vi "Red Pitaya OO Control.vi"(8 "Error In":errorcluster, 10 "Server port":u16=1002, 11 "Server address":string="192.168.1.100") -> (0 "Error Out":errorcluster)   [LabVIEW 2015]
uses:
  Mode.ctl
  Red Pitaya Parameters.ctl
  RP Core/RP Communicator/RP Communicator.lvclass
  RP Core/RP Communicator/RP Communicator.lvclass/RP Communicator.ctl
  RP Status Offsets.ctl
  RP Command.ctl
  RP Config Offsets.ctl
  RP Core/RP Communicator/Write Client type.vi
panel:
  in  "Controls":enum32{"Basic", "Advanced"}(tab)=enum."Advanced"
  out "X&Y":cluster{i32, i32}(graph)
  in  "Parameters":T1={"Ranges"=[0.0001, 0.01], "Output frequency 1"=15625000.0, "Output frequency 2"=50000.0, "Pre-trigger samples"=-100000, "Post-trigger samples"=11534336, "Desimation rate"=1, "Delayed start"=571428} {"Delayed start" format="0x%x (%d)"; "Post-trigger samples" format="0x%x (%d)"; "Pre-trigger samples" format="0x%x (%d)"; "Output frequency 2" format="%#_6p"; "Output frequency 1" format="%#_6p"; "Ranges" format="%#_12p"}
  out "CPU Temperature":dbl(slide)=48.847186279148 scale=0.0..100.0
  out "Y":i32=1717987 format="0x%x (%d)"
  out "X":i32=1717987 format="0x%x (%d)"
  in  "Read XY":bool
  in  "Trigger pos acuracy":i32=1
  in  "Signal bits":i32=14
  in  "Read Temperature":bool
  in  "Read trigger":bool=TRUE
  in  "Auto-save file":bool
  in  "Samples to read":u64=67108864 format="0x%x (%d)"
  in  "Record":bool
  out "Temperature Chart":dbl(graph)=48.847186279148
  out "bytes written":i32=8
  in  "Status":bool
  out "Status response":u32=1 format="0x%x (%d)"
  out "element":u32
  in  "Status offset":u64=12
  out "Phase increment 1":u64=1717987 format="0x%x (%d)"
  in  "Read":bool
  in  "Send \"Connect client\"":bool=TRUE
  in  "Bytes per sample":i32=4
  out "Is Red Pitaya?":bool
  out "Logic tag out":u16
  out "IDN response":u32=1 format="0x%x (%d)"
  in  "Read subset":bool
  out "Data File  Path":path
  out "Trigger state":bool
  in  "Trigger":bool
  in  "Arm":bool
  out "Phase  Graph":u32[](graph)
  in  "Mode":T2=enum."Current-Voltage"
  out "Waveform Graph":sgl[][](graph)
  in  "Stop Server":bool
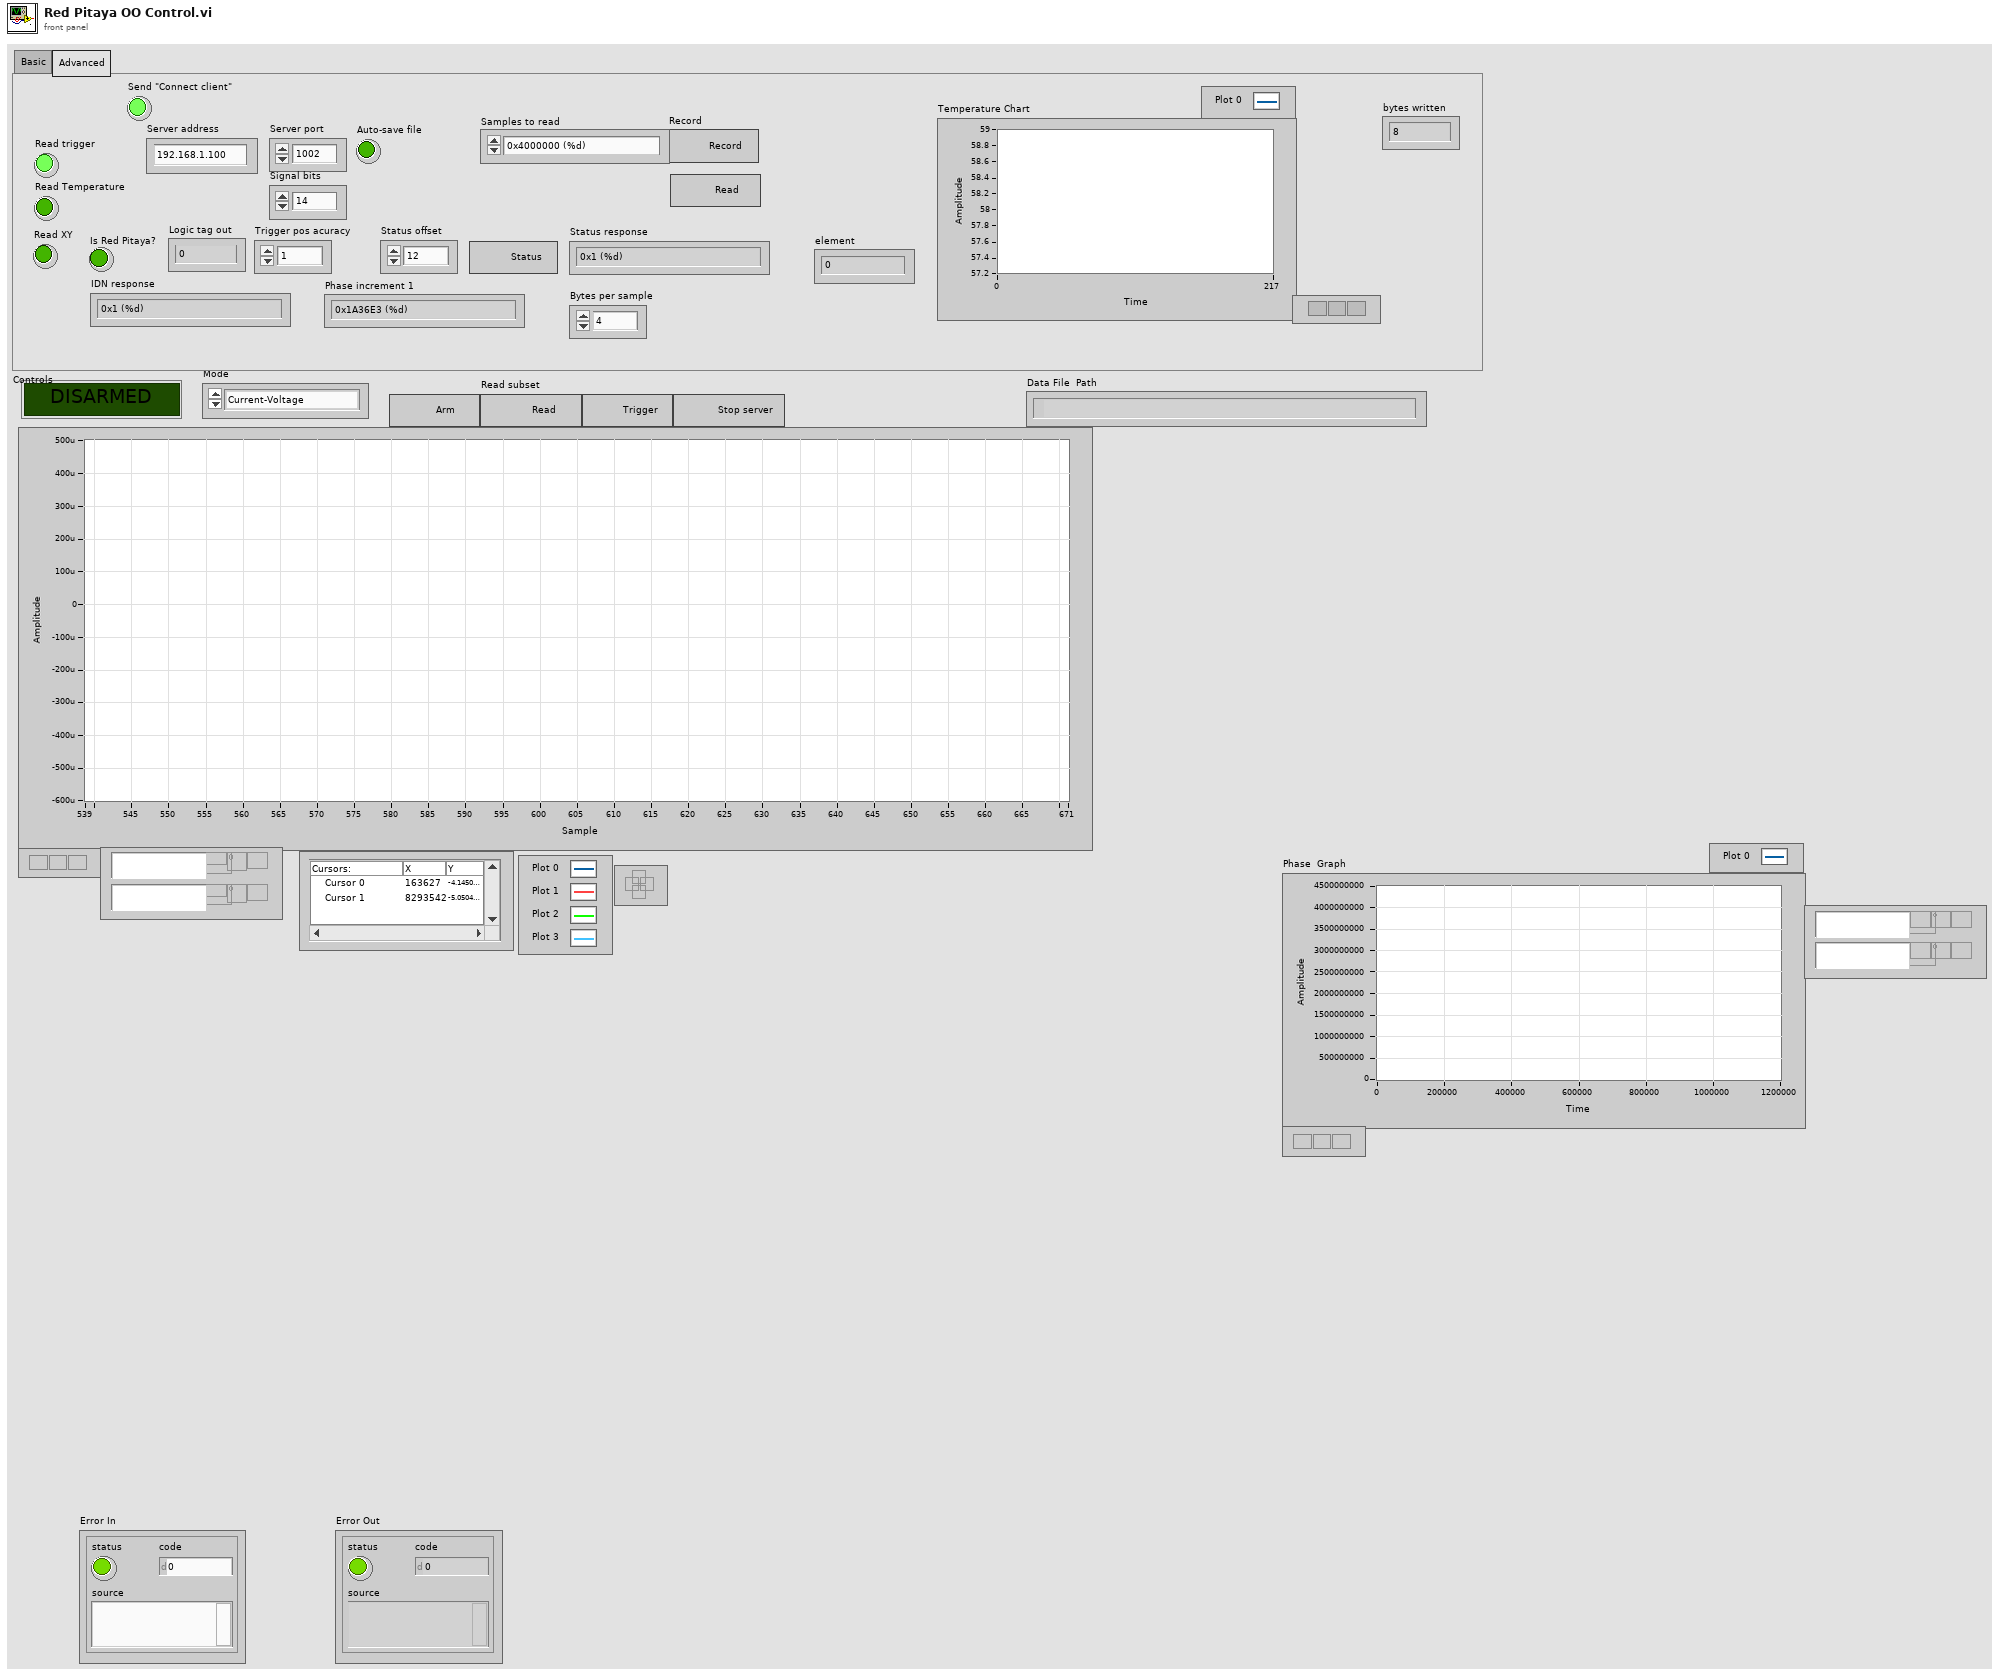
[diagram p1: front panel]
types:
  T1 = typedef "Red Pitaya Parameters.ctl" = cluster{"Ranges":dbl[], "Output frequency 1":dbl, "Output frequency 2":dbl, "Pre-trigger samples":i32, "Post-trigger samples":u64, "Desimation rate":u64, "Delayed start":u64}
  T2 = typedef "Mode.ctl" = enum16{"Filter", "Lockin test", "Snapshot test", "Digitizer", "Current-Voltage"}
  T3 = typedef "RP Command.ctl" = enum16{"Reset", "Read IDN", "Stop server", "Get status", "Get temperature", "Connect client", "Arm", "Software trigger", "Get whole buffer", "Get chunk", "System call", "Get config", "Set config", "Recieve data", "Play pattern", "Transmit data"}
  T4 = typedef "RP Status Offsets.ctl" = u16
  T5 = typedef "RP Config Offsets.ctl" = u16
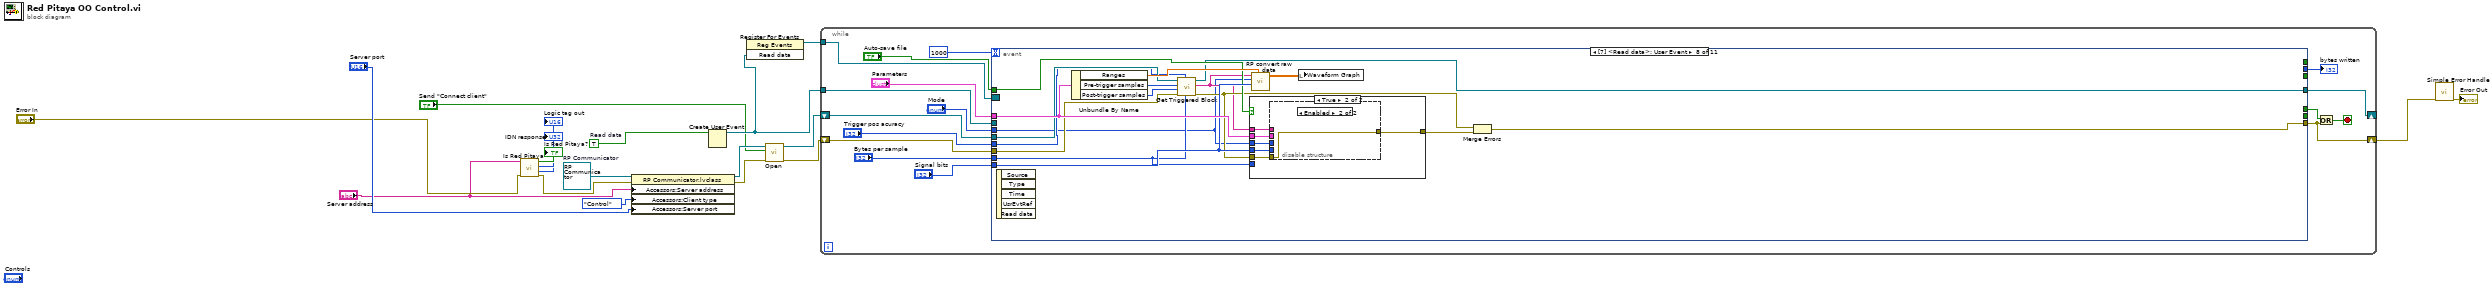
[diagram p0: block diagram]
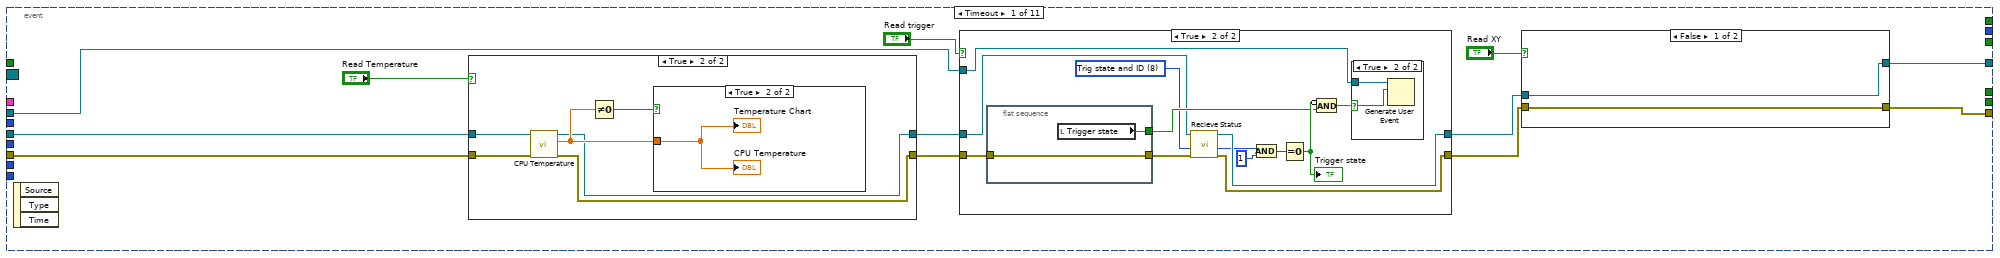
[diagram p2: hidden frame]
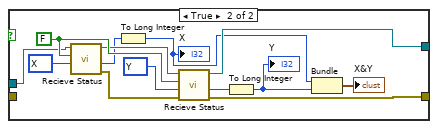
[diagram p3: hidden frame]
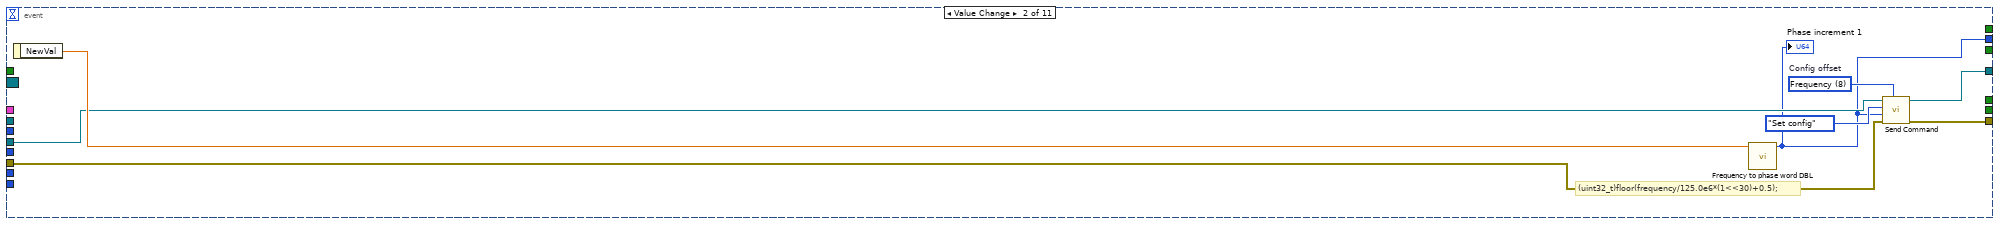
[diagram p8: hidden frame]
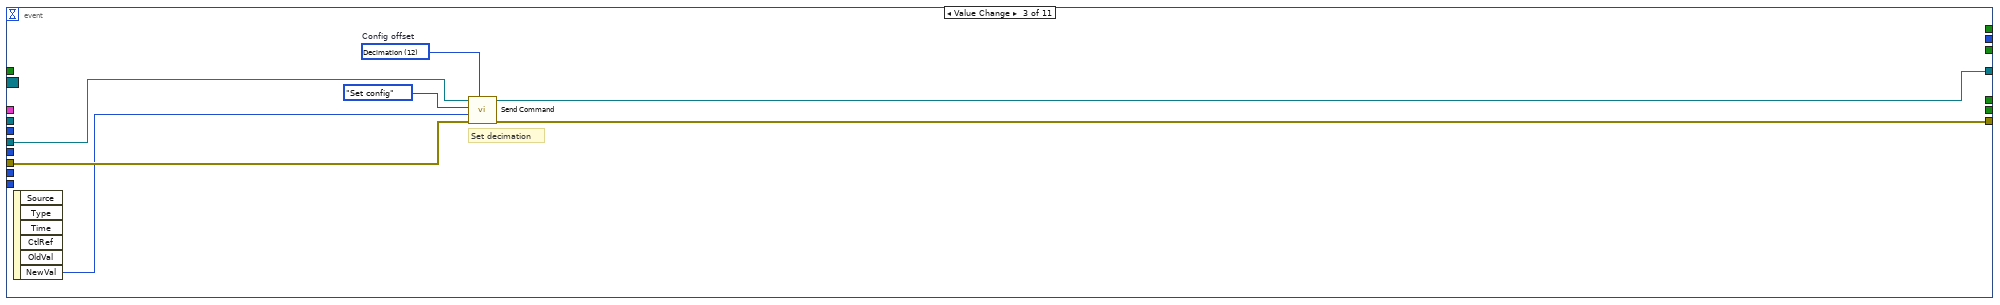
[diagram p9: hidden frame]
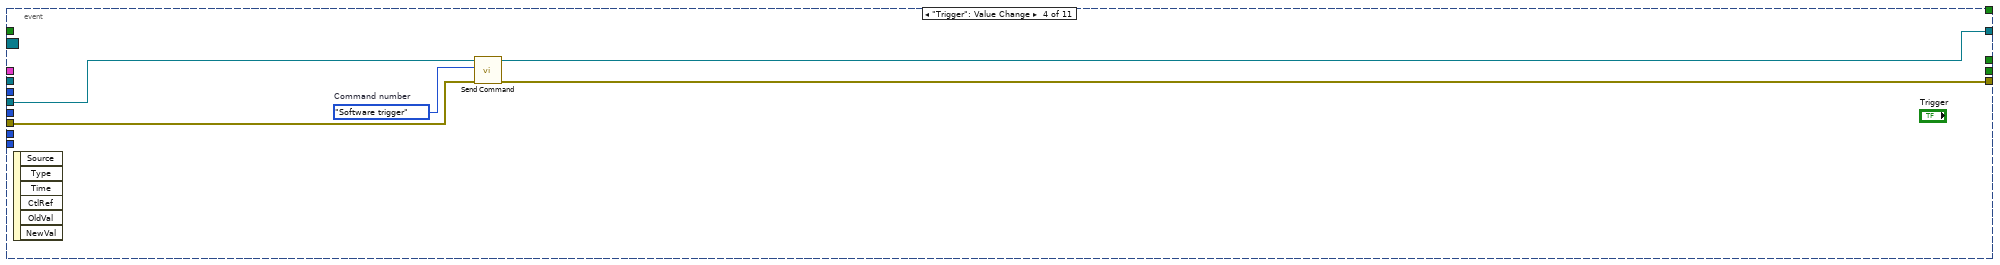
[diagram p10: hidden frame]
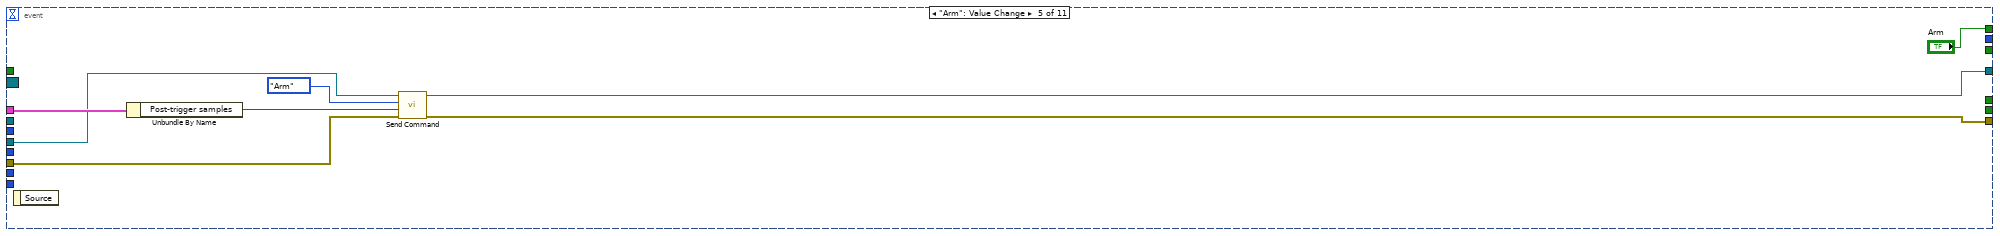
[diagram p11: hidden frame]
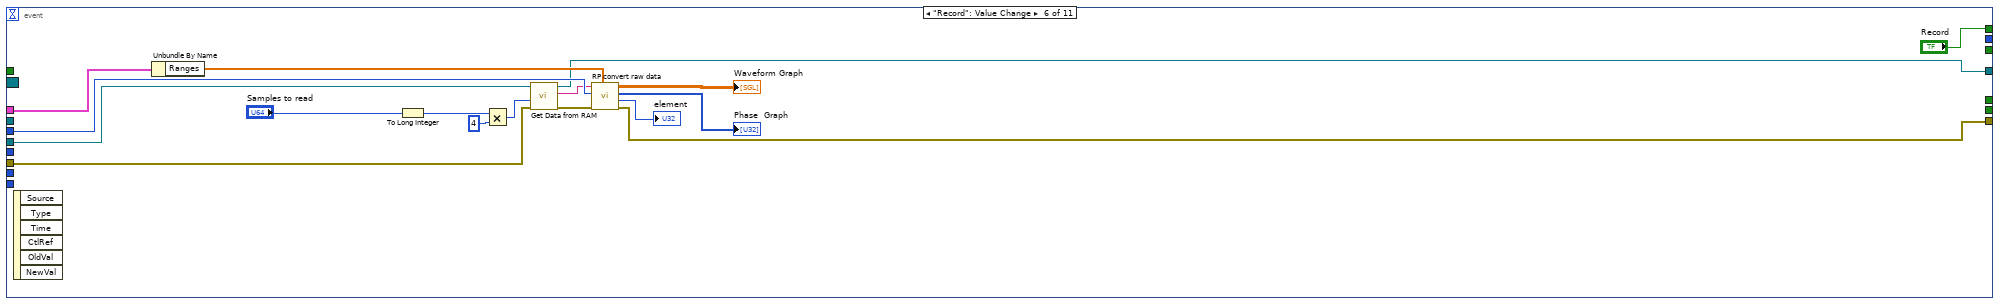
[diagram p12: hidden frame]
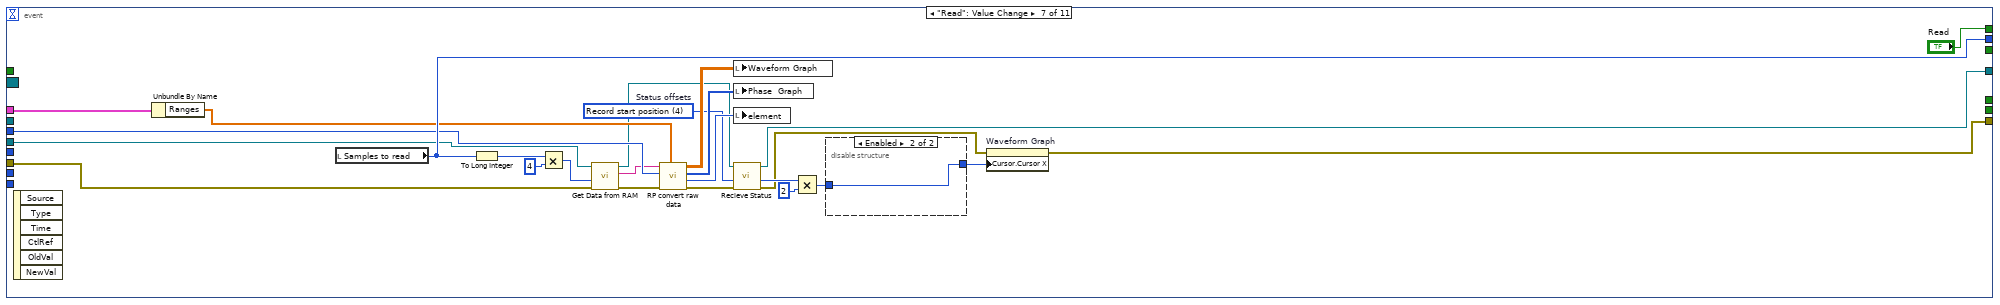
[diagram p13: hidden frame]
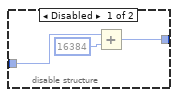
[diagram p14: hidden frame]
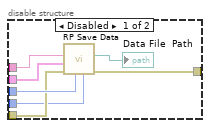
[diagram p16: hidden frame]
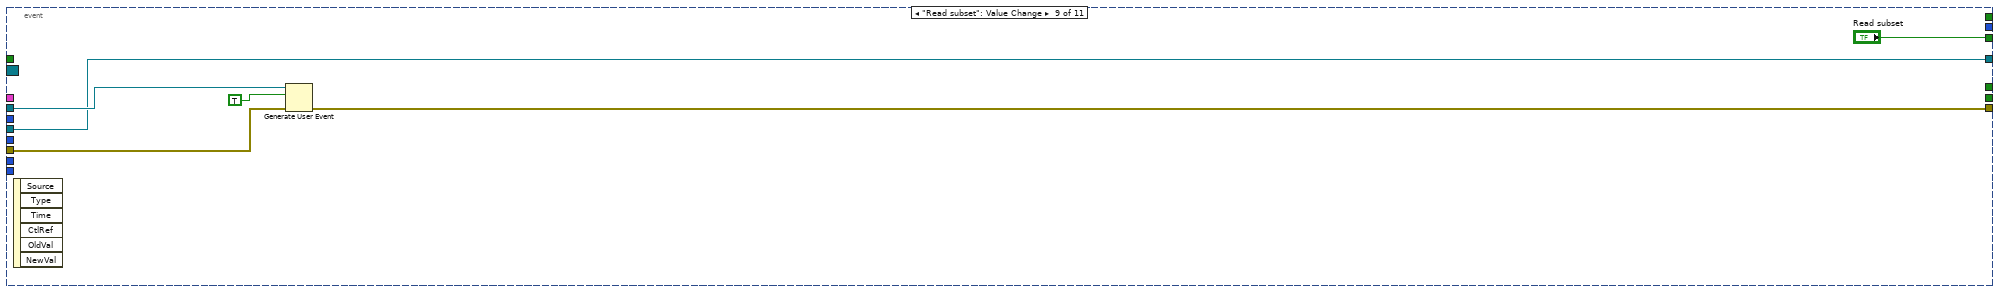
[diagram p17: hidden frame]
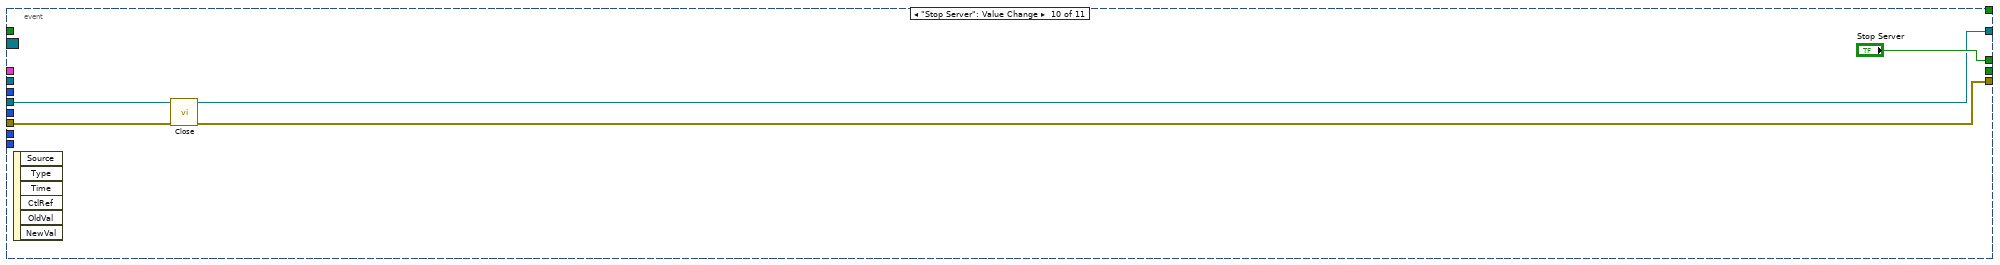
[diagram p18: hidden frame]
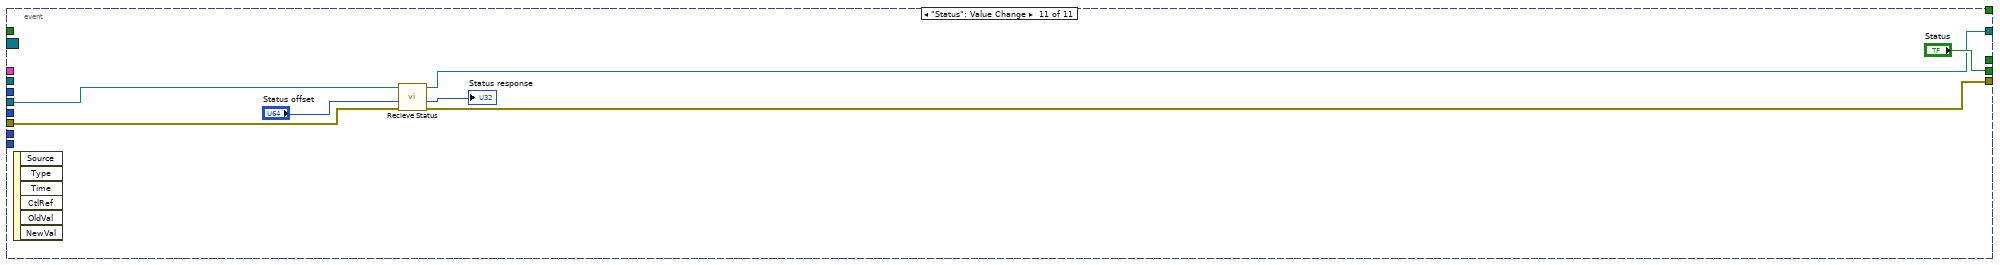
[diagram p19: hidden frame]
diagram:
  w13 = refnum<class "RP Communicator.lvclass"> refnum  # RP Communicator
  w17 = TRUE  # Read data
  n1 = call "Is Red Pitaya.vi"("Error In"="Error In", "Server address"="Server address") -> ("Error Out"=w5:errorcluster, "Logic tag out"=→"Logic tag out":u16, "IDN response"=→"IDN response":u32, "Red Pitaya"=→"Is Red Pitaya?":bool)  [unwired: 5 in, 1 out]
  n2 = property class="RP Communicator.lvclass"(reference=w13, error in=w5, "Accessors:Server address"="Server address", "Accessors:Client type"=enum16{"Control", "Reciever", "Transmitter"}."Control" ("Client type"), "Accessors:Server port"="Server port") -> (reference out=w14:refnum<class "RP Communicator.lvclass">, error out=w11:errorcluster)
  n3 = Create User Event(user event datatype=w17) -> (user event=w15:refnum<user-event>)  [unwired: 1 in, 1 out]
  n4 = register-events(w15) -> (reference out=w16:refnum<event-registration>)  [unwired: 2 in, 1 out]
  n5 = call-dynamic "Open.vi"("error in (no error)"=w11, "Send \"Connect client\""="Send \"Connect client\"", "RP Communicator in"=w14) -> ("error out"=w9:errorcluster, "RP Communicator out"=w10:refnum<class "RP Communicator.lvclass">)  [unwired: 7 in]
  n6 = while {
    shift-right: [w33] -> w19
    shift-left: w9 -> [w35]
    tunnel: w16 -> [w24]
    tunnel: w15 -> [w23]
    shift-right: [w21] -> _
    shift-left: w10 -> [w22]
    stop <- w31 stop-if-true
    n7 = event shown="[7] <Read data>: User Event" {
      selector: w24 -> [_ _ _ _ _ _ _ _ _ _ _]
      dyn-events: _ -> [_ _ _ _ _ _ _ _ _ _ _]
      timeout: 1000 -> [_ _ _ _ _ _ _ _ _ _ _]
      tunnel: w35 -> [w46 w93 w101 w107 w113 w123 w145 w173 w199 w204 w210]
      tunnel: [w42 w94 w102 w108 w112 w131 w159 w181 w198 w203 w209] -> w33
      tunnel: [_ _ _ _ _ _ _ _ _ "Stop Server" _] -> w32
      tunnel: [_ _ _ _ _ _ _ _ _ _ "Status"] -> _
      tunnel: [_ w91 _ _ _ _ w156 _ _ _ _] -> w34
      tunnel: [_ _ _ _ "Arm" "Record" "Read" _ _ _ _] -> _
      tunnel: "Mode" -> [_ _ _ _ _ w128 w149 w165 _ _ _]
      tunnel: "Parameters" -> [_ _ _ _ w117 w127 w148 w179 _ _ _]
      tunnel: "Signal bits" -> [_ _ _ _ _ _ _ w177 _ _ _]
      tunnel: "Trigger pos acuracy" -> [_ _ _ _ _ _ _ w167 _ _ _]
      tunnel: "Auto-save file" -> [_ _ _ _ _ _ _ w175 _ _ _]
      tunnel: [_ _ _ _ _ _ _ _ "Read subset" _ _] -> _
      tunnel: w23 -> [w40 _ _ _ _ _ _ _ w201 _ _]
      tunnel: w22 -> [w39 w96 w99 w106 w116 w125 w146 w174 w197 w206 w213]
      tunnel: [w36 w95 w103 w109 w111 w120 w136 w172 w197 w205 w208] -> w21
      tunnel: "Bytes per sample" -> [_ _ _ _ _ _ _ w166 _ _ _]
      event Timeout {
        n8 = event-data() -> ()  [unwired: 1 in, 3 out]
        n9 = case shown="True" "Read Temperature" {
          tunnel: w46 -> [w83 w87]
          tunnel: [w83 w85] -> w44
          tunnel: w39 -> [w82 w88]
          tunnel: [w82 w84] -> w38
          frame False {
          }
          frame True {
            n10 = call-dynamic "CPU Temperature.vi"("error in (no error)"=w87, "RP Communicator in"=w88) -> ("error out"=w85:errorcluster, "CPU Temperature"=w86:dbl, "RP Communicator out"=w84:refnum<class "RP Communicator.lvclass">)  [unwired: 7 in]
            n11 = Not Equal To 0?(x=w86) -> (x != 0?=w89:bool)
            n12 = case shown="True" w89 {
              tunnel: w86 -> [_ w90]
              frame False {
              }
              frame True {
                "CPU Temperature" <- w90
                "Temperature Chart" <- w90
              }
            }
          }
        }
        n13 = case shown="True" "Read trigger" {
          tunnel: w44 -> [w64 w75]
          tunnel: [w64 w68] -> w43
          tunnel: w40 -> [_ w71]
          tunnel: w38 -> [w63 w70]
          tunnel: [w63 w66] -> w37
          frame False {
          }
          frame True {
            w67 = T4 8 items=["Writer address"=0, "Record start position"=4, "Trig state and ID"=8, "Phase"=12, "Y"=16, "X"=20, "RxFIFO counter"=24, "TxFIFO counter"=28] ("Status offsets")
            n14 = flat-sequence {
              tunnel: w75 -> [w81]
              tunnel: [w81] -> w69
              tunnel: [w80] -> w73
              frame #0 {
                n15 = local read "Trigger state"() -> (w80:bool)
              }
            }
            n16 = call-dynamic "Recieve Status.vi"("error in (no error)"=w69, "Status offset"=w67, "RP Communicator in"=w70) -> ("error out"=w68:errorcluster, "Status response"=w65:u32, "RP Communicator out"=w66:refnum<class "RP Communicator.lvclass">)  [unwired: 6 in]
            n17 = And(x=w65, y=u32 1) -> (x .and. y?=w76:u32)
            n18 = Equal To 0?(x=w76) -> (x = 0?=w74:bool)
            "Trigger state" <- w74
            n19 = Compound Arithmetic op=AND(invert w74, w73) -> (w72:bool)
            n20 = case shown="True" w72 {
              selector: w72 -> [_ w78]
              tunnel: w71 -> [_ w79]
              frame False {
              }
              frame True {
                n21 = Generate User Event(user event=w79, event data cluster=w78) -> ()  [unwired: 2 in, 2 out]
              }
            }
          }
        }
        n22 = case shown="False" "Read XY" {
          tunnel: w43 -> [w49 _]
          tunnel: [w49 w50] -> w42
          tunnel: w37 -> [w48 w54]
          tunnel: [w48 w53] -> w36
          frame False {
          }
          frame True {
            w59 = T4 20 items=["Writer address"=0, "Record start position"=4, "Trig state and ID"=8, "Phase"=12, "X"=16, "Y"=20, "RxFIFO counter"=24, "TxFIFO counter"=28] ("Status offset")
            w56 = T4 16 items=["Writer address"=0, "Record start position"=4, "Trig state and ID"=8, "Phase"=12, "X"=16, "Y"=20, "RxFIFO counter"=24, "TxFIFO counter"=28] ("Status offset")
            w60 = FALSE ("Read config instead")
            n23 = call-dynamic "Recieve Status.vi"("Status offset"=w56, "Read config instead"=w60, "RP Communicator in"=w54) -> ("error out"=w57:errorcluster, "Status response"=w55:u32, "RP Communicator out"=w58:refnum<class "RP Communicator.lvclass">)  [unwired: 6 in]
            n24 = To Long Integer(number=w55) -> (32bit integer=w51:i32)
            "X" <- w51
            n25 = call-dynamic "Recieve Status.vi"("error in (no error)"=w57, "Status offset"=w59, "Read config instead"=w60, "RP Communicator in"=w58) -> ("error out"=w50:errorcluster, "Status response"=w61:u32, "RP Communicator out"=w53:refnum<class "RP Communicator.lvclass">)  [unwired: 5 in]
            n26 = To Long Integer(number=w61) -> (32bit integer=w52:i32)
            "Y" <- w52
            n27 = Bundle(w51, w52) -> (→"X&Y":cluster{i32, i32})  [unwired: 1 in]
          }
        }
      }
      event Value Change {
        w97 = T5 8 items=["Config flags"=0, "Record length"=4, "Frequency"=8, "Decimation"=12, "LED"=16, "DDS delay"=28]  # Config offset
        # "(uint32_t)floor(frequency/125.0e6*(1<<30)+0.5);"
        n28 = event-data() -> ("NewVal"=w98:dbl)  [unwired: 1 in]
        n29 = call "Frequency to phase word DBL.vi"("Frequency"=w98) -> ("Phase word"=w91:u64)  [unwired: 10 in]
        "Phase increment 1" <- w91
        n30 = call-dynamic "Send Command.vi"("Config offset"=w97, "error in (no error)"=w93, "Command payload"=w91, "Command number"=RP_Command."Set config", "RP Communicator in"=w96) -> ("error out"=w94:errorcluster, "RP Communicator out"=w95:refnum<class "RP Communicator.lvclass">)  [unwired: 5 in]
      }
      event Value Change {
        w105 = T5 12 items=["Config flags"=0, "Record length"=4, "Frequency"=8, "Decimation"=12, "LED"=16]  # Config offset
        # "Set decimation"
        n31 = event-data() -> ("NewVal"=w100:u64)  [unwired: 1 in, 5 out]
        n32 = call-dynamic "Send Command.vi"("Config offset"=w105, "error in (no error)"=w101, "Command payload"=w100, "Command number"=RP_Command."Set config", "RP Communicator in"=w99) -> ("error out"=w102:errorcluster, "RP Communicator out"=w103:refnum<class "RP Communicator.lvclass">)  [unwired: 5 in]
      }
      event "Trigger": Value Change {
        w110 = RP_Command."Software trigger"  # Command number
        n33 = event-data() -> ()  [unwired: 1 in, 6 out]
        n34 = call-dynamic "Send Command.vi"("error in (no error)"=w107, "Command number"=w110, "RP Communicator in"=w106) -> ("error out"=w108:errorcluster, "RP Communicator out"=w109:refnum<class "RP Communicator.lvclass">)  [unwired: 7 in]
      }
      event "Arm": Value Change {
        n35 = event-data() -> ()  [unwired: 1 in, 1 out]
        n36 = Unbundle By Name(w117) -> ("Post-trigger samples"=w114:u64)
        n37 = call-dynamic "Send Command.vi"("error in (no error)"=w113, "Command payload"=w114, "Command number"=RP_Command."Arm", "RP Communicator in"=w116) -> ("error out"=w112:errorcluster, "RP Communicator out"=w111:refnum<class "RP Communicator.lvclass">)  [unwired: 6 in]
      }
      event "Record": Value Change {
        n38 = event-data() -> ()  [unwired: 1 in, 6 out]
        n39 = Unbundle By Name(w127) -> ("Ranges"=w126:dbl[])
        n40 = To Long Integer(number="Samples to read") -> (32bit integer=w133:i32)
        n41 = Multiply(x=w133, y=4) -> (x*y=w119:i32)
        n42 = call-dynamic "Get Data from RAM.vi"("error in (no error)"=w123, "End offset"=w119, "RP Communicator in"=w125) -> ("error out"=w122:errorcluster, "data out"=w121:string, "RP Communicator out"=w120:refnum<class "RP Communicator.lvclass">)  [unwired: 6 in]
        n43 = call "RP convert raw data.vi"("Max Volts"=w126, "Error In"=w122, "Format"=w128, "data stream"=w121) -> ("Error Out"=w131:errorcluster, "element"=→"element":u32, "phase out"=→"Phase  Graph":u32[], "data out"=→"Waveform Graph":sgl[][])  [unwired: 4 in]
      }
      event "Read": Value Change {
        w140 = T4 4 items=["Writer address"=0, "Record start position"=4, "Trig state and ID"=8, "Phase"=12, "Y"=16, "X"=20, "RxFIFO counter"=24, "TxFIFO counter"=28]  # Status offsets
        n44 = event-data() -> ()  [unwired: 1 in, 6 out]
        n45 = Unbundle By Name(w148) -> ("Ranges"=w147:dbl[])
        n46 = local read "Samples to read"() -> (w156:u64)
        n47 = To Long Integer(number=w156) -> (32bit integer=w157:i32)
        n48 = Multiply(x=w157, y=4) -> (x*y=w144:i32)
        n49 = call-dynamic "Get Data from RAM.vi"("error in (no error)"=w145, "End offset"=w144, "RP Communicator in"=w146) -> ("error out"=w142:errorcluster, "data out"=w143:string, "RP Communicator out"=w141:refnum<class "RP Communicator.lvclass">)  [unwired: 6 in]
        n50 = call "RP convert raw data.vi"("Max Volts"=w147, "Error In"=w142, "Format"=w149, "data stream"=w143) -> ("Error Out"=w139:errorcluster, "element"=w153:u32, "phase out"=w154:u32[], "data out"=w155:sgl[][])  [unwired: 4 in]
        n51 = local write "Waveform Graph"(w155) -> ()
        n52 = local write "Phase  Graph"(w154) -> ()
        n53 = local write "element"(w153) -> ()
        n54 = call-dynamic "Recieve Status.vi"("error in (no error)"=w139, "Status offset"=w140, "RP Communicator in"=w141) -> ("error out"=w137:errorcluster, "Status response"=w138:u32, "RP Communicator out"=w136:refnum<class "RP Communicator.lvclass">)  [unwired: 6 in]
        n55 = Multiply(x=w138, y=u32 2) -> (x*y=w151:u32)
        n56 = disable-structure shown="Enabled" {
          disable-tunnel: w151 -> [w163 w164]
          disable-tunnel: [w161 w164] -> w150
          frame Disabled {
            n57 = Add(x=w163, y=16384) -> (x+y=w161:u32)
          }
          frame Enabled {
          }
        }
        n58 = property on="Waveform Graph" class="WFGraph (strict)"(error in=w137, "Cursor.Cursor X"=w150) -> (error out=w159:errorcluster)  [unwired: 1 in, 1 out]
      }
      event User Event {
        n59 = event-data() -> ()  [unwired: 1 in, 5 out]
        n60 = Unbundle By Name(w179) -> ("Ranges"=w178:dbl[], "Pre-trigger samples"=w169:i32, "Post-trigger samples"=w168:u64)
        n61 = call-dynamic "Get Triggered Block.vi"("Bytes per sample"=w166, "Samples per trigger increment"=w167, "error in (no error)"=w173, "Post-trigger samples"=w168, "Pre-trigger samples"=w169, "RP Communicator in"=w174) -> ("error out"=w171:errorcluster, "data out"=w170:string, "RP Communicator out"=w172:refnum<class "RP Communicator.lvclass">)  [unwired: 3 in]
        n62 = case shown="True" w175 {
          tunnel: w171 -> [w182 w185]
          tunnel: w170 -> [_ w187]
          tunnel: [w182 w183] -> w180
          tunnel: w179 -> [_ w188]
          tunnel: w165 -> [_ w186]
          tunnel: w177 -> [_ w184]
          tunnel: w166 -> [_ _]
          frame False {
          }
          frame True {
            n63 = disable-structure shown="Enabled" {
              disable-tunnel: w188 -> [w195 _]
              disable-tunnel: w187 -> [w194 _]
              disable-tunnel: w186 -> [w193 _]
              disable-tunnel: w185 -> [w192 w196]
              disable-tunnel: w184 -> [w191 _]
              disable-tunnel: [w190 w196] -> w183
              frame Disabled {
                n64 = call "RP Save Data.vi"("Signal bits"=w191, "Mode"=w193, "Error In"=w192, "Parameters"=w195, "Data stream"=w194) -> ("Error Out"=w190:errorcluster, "Data File  Path"=→"Data File  Path":path)  [unwired: 3 in, 2 out]
              }
              frame Enabled {
              }
            }
          }
        }
        n65 = call "RP convert raw data.vi"("Max Volts"=w178, "Signal bits"=w177, "Format"=w165, "data stream"=w170) -> ("data out"=w176:sgl[][])  [unwired: 4 in, 3 out]
        n66 = local write "Waveform Graph"(w176) -> ()
        n67 = Merge Errors(w171, w180) -> (w181:errorcluster)
      }
      event "Read subset": Value Change {
        n68 = event-data() -> ()  [unwired: 1 in, 6 out]
        n69 = Generate User Event(user event=w201, event data cluster=TRUE, error in=w199) -> (error out=w198:errorcluster)  [unwired: 1 in, 1 out]
      }
      event "Stop Server": Value Change {
        n70 = event-data() -> ()  [unwired: 1 in, 6 out]
        n71 = call-dynamic "Close.vi"("error in (no error)"=w204, "RP Communicator in"=w206) -> ("error out"=w203:errorcluster, "RP Communicator out"=w205:refnum<class "RP Communicator.lvclass">)  [unwired: 8 in]
      }
      event "Status": Value Change {
        n72 = event-data() -> ()  [unwired: 1 in, 6 out]
        n73 = call-dynamic "Recieve Status.vi"("error in (no error)"=w210, "Status offset"="Status offset", "RP Communicator in"=w213) -> ("error out"=w209:errorcluster, "Status response"=→"Status response":u32, "RP Communicator out"=w208:refnum<class "RP Communicator.lvclass">)  [unwired: 6 in]
      }
    }
    "bytes written" <- w34
    n74 = Or(x=w32, y=w33) -> (x .or. y?=w31:bool)
  }
  n75 = call <vilib>:"Simple Error Handler.vi"("error in (no error)"=w19) -> ("error out"=→"Error Out":errorcluster)  [unwired: 4 in, 4 out]
